vi "set output trigger polarity.vi"(8 "error in (no error)":errorcluster, 11 "DAQOrcaFlash in":refnum<class "DAQOrcaFlash.lvclass">) -> (0 "error out":errorcluster, 3 "DAQOrcaFlash out":refnum<class "DAQOrcaFlash.lvclass">)   [LabVIEW 2012, in "DAQOrcaFlash.lvclass"]
uses:
  DAQOrcaFlash.lvclass
  DAQOrcaFlash.lvclass/DAQOrcaFlash.ctl
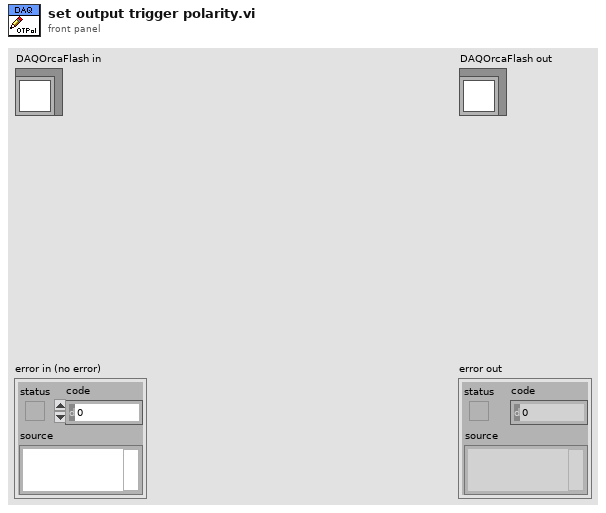
[diagram p1: front panel]
types:
  T1 = typedef "DAQOrcaFlash.lvclass/connector.ctl" = enum32{"1", "2", "3"}
  T2 = typedef "DAQOrcaFlash.lvclass/trigger_polarity.ctl" = sgl
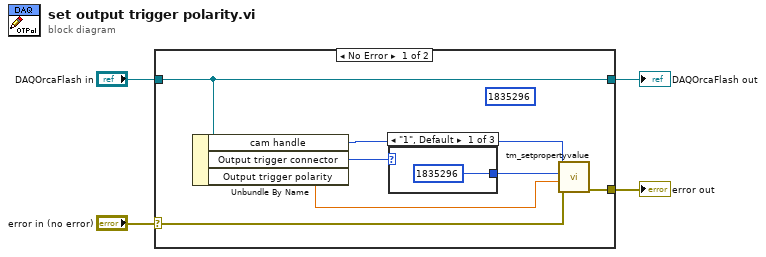
[diagram p0: block diagram]
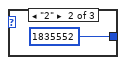
[diagram p2: hidden frame]
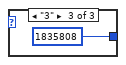
[diagram p3: hidden frame]
diagram:
  n1 = case shown="No Error" "error in (no error)" {
    selector: "error in (no error)" -> [w7 w16]
    tunnel: [w6 w16] -> w3
    tunnel: [w11 w15] -> w1
    tunnel: "DAQOrcaFlash in" -> [w11 w15]
    frame No Error {
      (unwired) 1835296
      n2 = Unbundle By Name(w11) -> ("cam handle"=w5:u32, "Output trigger connector"=w10:T1, "Output trigger polarity"=w8:T2)
      n3 = case shown="\"1\", Default" w10 {
        tunnel: [u32 1835296 u32 1835552 u32 1835808] -> w9
        frame "1", Default {
        }
        frame "2" {
        }
        frame "3" {
        }
      }
      n4 = call <userlib>:"tm_setpropertyvalue.vi"("error in (no error)"=w7, "Value in"=w8, "Property ID"=w9, "Handle in"=w5) -> ("error out"=w6:errorcluster)  [unwired: 6 in, 1 out]
    }
    frame Error {
    }
  }
  "error out" <- w3
  "DAQOrcaFlash out" <- w1
